vi "Witness Read.vi"(1 "address string":string) -> (0 "Field":dbl format="%.4f")   [LabVIEW 2010]
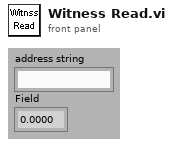
[diagram p1: front panel]
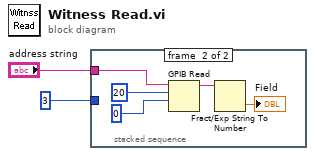
[diagram p0: block diagram]
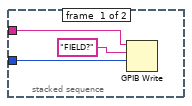
[diagram p2: hidden frame]
diagram:
  n1 = stacked-sequence {
    tunnel: "address string" -> [w4 w10]
    tunnel: i16 3 ("mode (0)") -> [w5 _]
    frame #0 {
      n2 = GPIB Write(0:w4, 1:"FIELD?" ("data"), 2:w5) -> ()  [unwired: 2 in, 2 out]
    }
    frame #1 {
      n3 = GPIB Read(0:w10, 1:20 ("byte count"), 2:i16 0 ("mode (0)")) -> (5:w7:string)  [unwired: 2 in, 2 out]
      n4 = Fract/Exp String To Number(string=w7) -> (number=→"Field":dbl)  [unwired: 3 in, 1 out]
    }
  }
